vi "Inside Circle.vi"(7 "Radius":dbl, 8 "y0":dbl, 9 "y":dbl, 10 "x0":dbl, 11 "x":dbl) -> (3 "Inside Circle":bool)   [LabVIEW 2010]
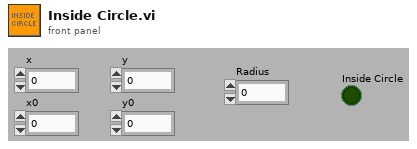
[diagram p1: front panel]
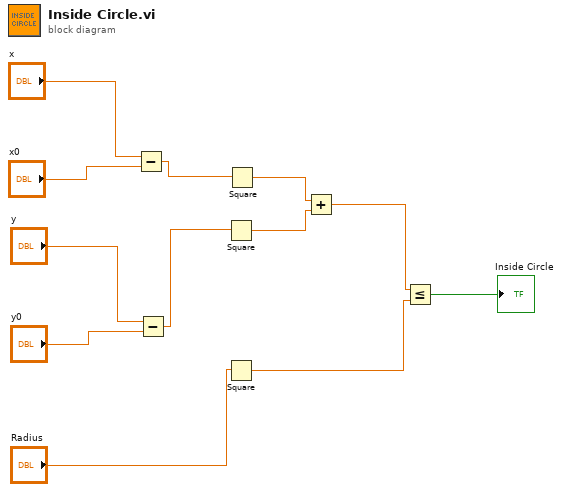
[diagram p0: block diagram]
diagram:
  n1 = Subtract(x="x", y="x0") -> (x-y=w10:dbl)
  n2 = Subtract(x="y", y="y0") -> (x-y=w7:dbl)
  n3 = Square(x=w7) -> (x^2=w5:dbl)
  n4 = Square(x="Radius") -> (x^2=w2:dbl)
  n5 = Square(x=w10) -> (x^2=w6:dbl)
  n6 = Add(x=w6, y=w5) -> (x+y=w4:dbl)
  n7 = Less Or Equal?(x=w4, y=w2) -> (x <= y?=→"Inside Circle":bool)
